vi "Launcher.vi"() -> ()   [LabVIEW 2020]
panel:
  in  "Exit":bool
  in  "Nuevo":bool
  in  "Stop":bool
  in  "Actores":u16(ring)
  in  "Tipo de Actor":enum16{""}(ring)
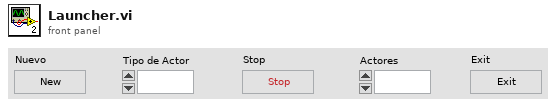
[diagram p1: front panel]
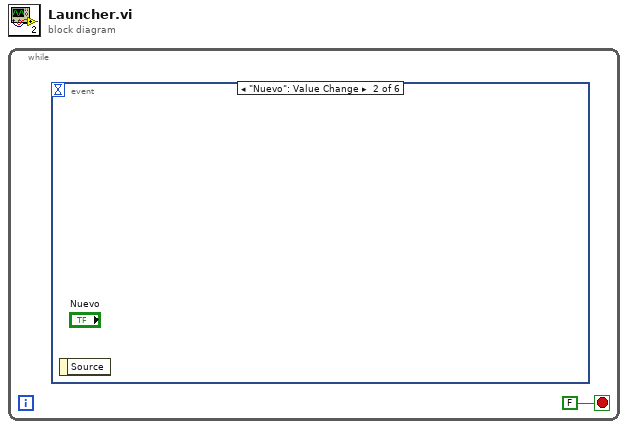
[diagram p0: block diagram]
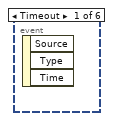
[diagram p2: hidden frame]
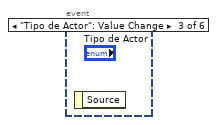
[diagram p3: hidden frame]
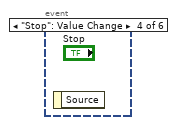
[diagram p4: hidden frame]
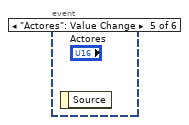
[diagram p5: hidden frame]
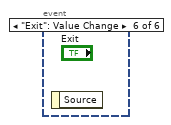
[diagram p6: hidden frame]
diagram:
  n1 = while {
    stop <- FALSE stop-if-true
    n2 = event shown="[1] \"Nuevo\": Value Change" {
      selector: _ -> [_ _ _ _ _ _]
      dyn-events: _ -> [_ _ _ _ _ _]
      timeout: _ -> [_ _ _ _ _ _]
      event Timeout {
        n3 = event-data() -> ()  [unwired: 1 in, 3 out]
      }
      event "Nuevo": Value Change {
        n4 = event-data() -> ()  [unwired: 1 in, 1 out]
      }
      event "Tipo de Actor": Value Change {
        n5 = event-data() -> ()  [unwired: 1 in, 1 out]
      }
      event "Stop": Value Change {
        n6 = event-data() -> ()  [unwired: 1 in, 1 out]
      }
      event "Actores": Value Change {
        n7 = event-data() -> ()  [unwired: 1 in, 1 out]
      }
      event "Exit": Value Change {
        n8 = event-data() -> ()  [unwired: 1 in, 1 out]
      }
    }
  }
